vi "VelStorageTF.vi"(8 "Int. Step (ms)":dbl=0.05, 9 "Retinal Slip":dbl, 11 "Leak cnt":dbl) -> (3 "Eye position":dbl)   [LabVIEW 2013]
doc: "Implements the Velocity storage's state space equations and integrate them via Euler Rule"
panel:
  # "State Space Representation"
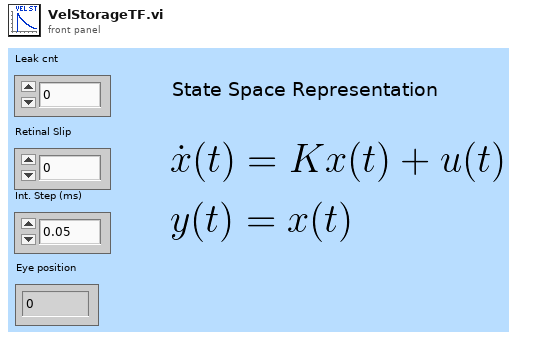
[diagram p1: front panel]
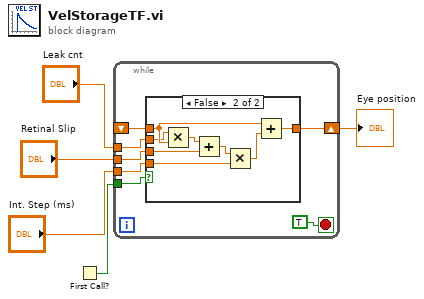
[diagram p0: block diagram]
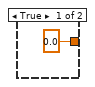
[diagram p2: hidden frame]
diagram:
  n1 = First Call?() -> (First Call?: T/F=w1:bool)
  n2 = while {
    tunnel: "Retinal Slip" -> [w12]
    tunnel: "Int. Step (ms)" -> [w9]
    tunnel: "Leak cnt" -> [w8]
    shift-right: [w11] -> w4
    shift-left: _ -> [w10]
    tunnel: w1 -> [w7]
    stop <- TRUE stop-if-true
    n3 = case shown="False" w7 {
      tunnel: w12 -> [_ w21]
      tunnel: [0.0 w20] -> w11
      tunnel: w10 -> [_ w19]
      tunnel: w9 -> [_ w17]
      tunnel: w8 -> [_ w15]
      frame True {
      }
      frame False {
        n4 = Multiply(x=w15, y=w19) -> (x*y=w14:dbl)
        n5 = Add(x=w14, y=w21) -> (x+y=w16:dbl)
        n6 = Multiply(x=w16, y=w17) -> (x*y=w18:dbl)
        n7 = Add(x=w19, y=w18) -> (x+y=w20:dbl)
      }
    }
  }
  "Eye position" <- w4
